vi "Grow info.vi"(1 "XRef":refnum<vi>, 2 "State In":T5) -> (0 "Grow Info":T1)   [LabVIEW 2012, in "ArrayDimension.xnode"]
uses:
  ArrayDimension.xnode
  State.ctl
  <vilib>/XNodeSupport/XNodeGrowInfo.ctl
  <vilib>/XNodeSupport/XNodeBounds.ctl
  <vilib>/XNodeSupport/XNodeInt.ctl
  <vilib>/XNodeSupport/XNodeBool.ctl
  <vilib>/XNodeSupport/NI_XNodeSupport.lvlib
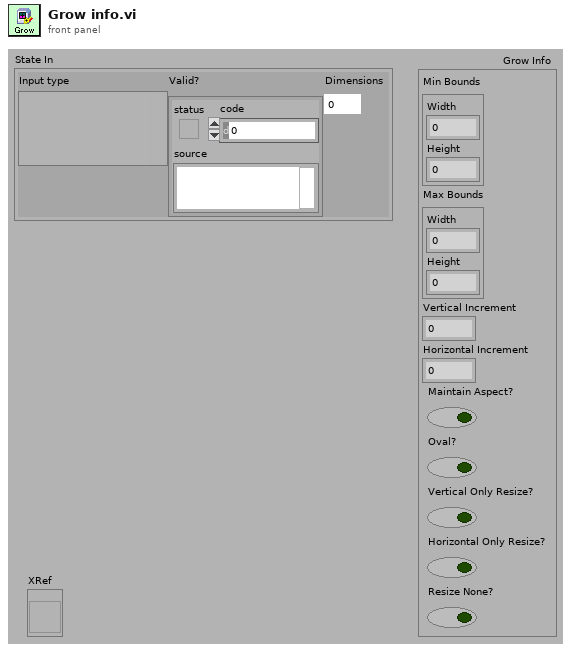
[diagram p1: front panel]
types:
  T1 = typedef "NI_XNodeSupport.lvlib/XNodeGrowInfo.ctl" = cluster{"Min Bounds":T2, "Max Bounds":T2, "Vertical Increment":T3, "Horizontal Increment":T3, "Maintain Aspect?":T4, "Oval?":T4, "Vertical Only Resize?":T4, "Horizontal Only Resize?":T4, "Resize None?":T4}
  T2 = typedef "NI_XNodeSupport.lvlib/XNodeBounds.ctl" = cluster{"Width":T3, "Height":T3}
  T3 = typedef "NI_XNodeSupport.lvlib/XNodeInt.ctl" = i32
  T4 = typedef "NI_XNodeSupport.lvlib/XNodeBool.ctl" = bool
  T5 = typedef "ArrayDimension.xnode/State.ctl" = cluster{"Input type":variant, "Valid?":errorcluster, "Dimensions":i32}
  T6 = cluster{"Min Bounds":T2, "Max Bounds":T2, "Vertical Increment":T3, "Horizontal Increment":T3, "Maintain Aspect?":T4, "Oval?":T4, "Vertical Only Resize?":T4, "Horizontal Only Resize?":T4, "Resize None?":T4}
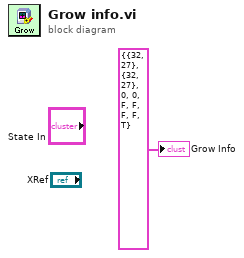
[diagram p0: block diagram]
diagram:
  "Grow Info" <- T6 {"Min Bounds"={"Width"=32, "Height"=27}, "Max Bounds"={"Width"=32, "Height"=27}, "Vertical Increment"=0, "Horizontal Increment"=0, "Maintain Aspect?"=FALSE, "Oval?"=FALSE, "Vertical Only Resize?"=FALSE, "Horizontal Only Resize?"=FALSE, "Resize None?"=TRUE} ("Grow Info")
